vi "dfd_Get Stopband Matrix (Even).vi"(7 "number of bands":i32=4, 9 "roll off":dbl, 11 "order":i32) -> (2 "Us":dbl[][](array[numeric]))   [LabVIEW 2017, in "NI_DigFilter_FilterBank.lvlib"]
uses:
  <vilib>/addons/Digital Filter Design/NI_DigFilter_FilterBank.lvlib
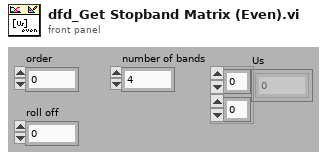
[diagram p1: front panel]
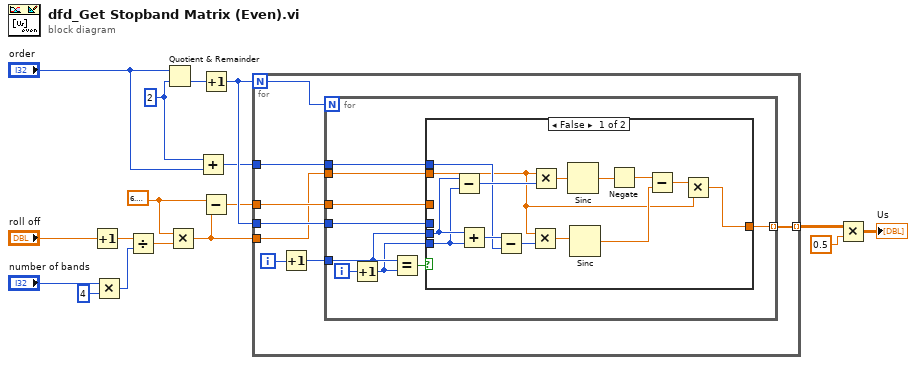
[diagram p0: block diagram]
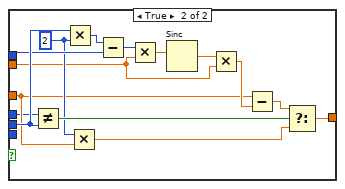
[diagram p2: hidden frame]
diagram:
  w16 = 6.283185307179586
  w11 = 2
  n1 = Increment(x="roll off") -> (x+1=w4:dbl)
  n2 = Multiply(x="number of bands", y=4) -> (x*y=w8:i32)
  n3 = Divide(x=w4, y=w8) -> (x/y=w3:dbl)
  n4 = Quotient & Remainder(x="order", y=w11) -> (floor(x/y)=w17:i32)  [unwired: 1 out]
  n5 = Multiply(x=w16, y=w3) -> (x*y=w9:dbl)
  n6 = Add(x=w11, y="order") -> (x+y=w10:i32)
  n7 = Increment(x=w17) -> (x+1=w14:i32)
  n8 = Subtract(x=w16, y=w9) -> (x-y=w13:dbl)
  n9 = for {
    N: w14 -> [w25]
    tunnel: w14 -> [w22]
    tunnel: w13 -> [w21]
    tunnel: w10 -> [w20]
    tunnel: w9 -> [w19]
    tunnel: [w18] -> w7 mode=indexing
    i -> [w24]
    n10 = Increment(x=w24) -> (x+1=w23:i32)
    n11 = for {
      N: w25 -> [_]
      tunnel: w23 -> [w31]
      tunnel: w22 -> [w32]
      tunnel: w21 -> [w30]
      tunnel: w20 -> [w29]
      tunnel: w19 -> [w28]
      tunnel: [w26] -> w18 mode=indexing
      i -> [w34]
      n12 = Increment(x=w34) -> (x+1=w27:i32)
      n13 = Equal?(x=w31, y=w27) -> (x = y?=w33:bool)
      n14 = case shown="False" w33 {
        tunnel: w32 -> [_ w51]
        tunnel: w31 -> [w46 w62]
        tunnel: w30 -> [_ w54]
        tunnel: w29 -> [w43 w60]
        tunnel: w28 -> [w35 w49]
        tunnel: [w36 w50] -> w26
        tunnel: w27 -> [w45 _]
        frame False {
          n15 = Subtract(x=w46, y=w45) -> (x-y=w47:i32)
          n16 = Add(x=w46, y=w45) -> (x+y=w44:i32)
          n17 = Subtract(x=w44, y=w43) -> (x-y=w41:i32)
          n18 = Multiply(x=w35, y=w41) -> (x*y=w42:dbl)
          n19 = Multiply(x=w35, y=w47) -> (x*y=w48:dbl)
          n20 = Sinc(1:w48) -> (0:w38:dbl)
          n21 = Sinc(1:w42) -> (0:w39:dbl)
          n22 = Negate(x=w38) -> (-x=w37:dbl)
          n23 = Subtract(x=w37, y=w39) -> (x-y=w40:dbl)
          n24 = Multiply(x=w40, y=w35) -> (x*y=w36:dbl)
        }
        frame True {
          w55 = 2
          n25 = Not Equal?(x=w51, y=w62) -> (x != y?=w63:bool)
          n26 = Multiply(x=w62, y=w55) -> (x*y=w61:i32)
          n27 = Multiply(x=w55, y=w54) -> (x*y=w52:dbl)
          n28 = Subtract(x=w61, y=w60) -> (x-y=w57:i32)
          n29 = Multiply(x=w57, y=w49) -> (x*y=w59:dbl)
          n30 = Sinc(1:w59) -> (0:w58:dbl)
          n31 = Multiply(x=w58, y=w49) -> (x*y=w56:dbl)
          n32 = Subtract(x=w54, y=w56) -> (x-y=w53:dbl)
          n33 = Select(t=w53, s=w63, f=w52) -> (s? t:f=w50:dbl)
        }
      }
    }
  }
  n34 = Multiply(x=w7, y=0.5) -> (x*y=→"Us":dbl[][])
